vi "Discover ALL VIs in Memory.vi"(5 "Show Progress (T)":bool=TRUE, 6 "Filtered Paths":path[](array[path]), 7 "Search Clones Up To":i32=100, 8 "error in":errorcluster, 9 "Globals?":bool=TRUE, 10 "File Extension Filters":string[](array[string]), 11 "Application in":refnum<vi>) -> (0 "error out":errorcluster, 1 "VIs (including clones)":string[](array[string]), 3 "Application out":refnum<vi>)   [LabVIEW 2013, in "LVTM.lvlib"]
uses:
  LVTM.lvlib
  Clone VIs FG Enum.ctl
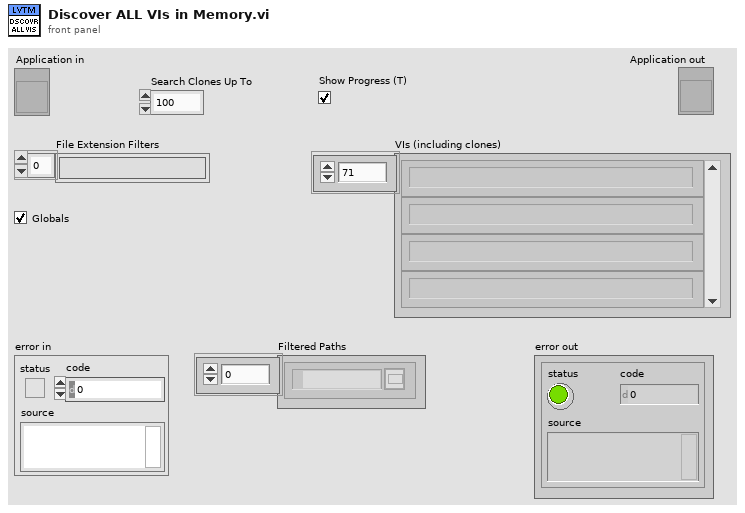
[diagram p1: front panel]
types:
  T1 = typedef "LVTM.lvlib/Clone VIs FG Enum.ctl" = enum16{"Get", "Get Active VIs", "Add VI"}
  T2 = enum32{"invalid VI type", "Standard VI", "Control VI", "Global VI", "Polymorphic VI", "Configuration VI", "SubSystem", "Facade VI", "Method VI", "Statechart Diagram VI"}
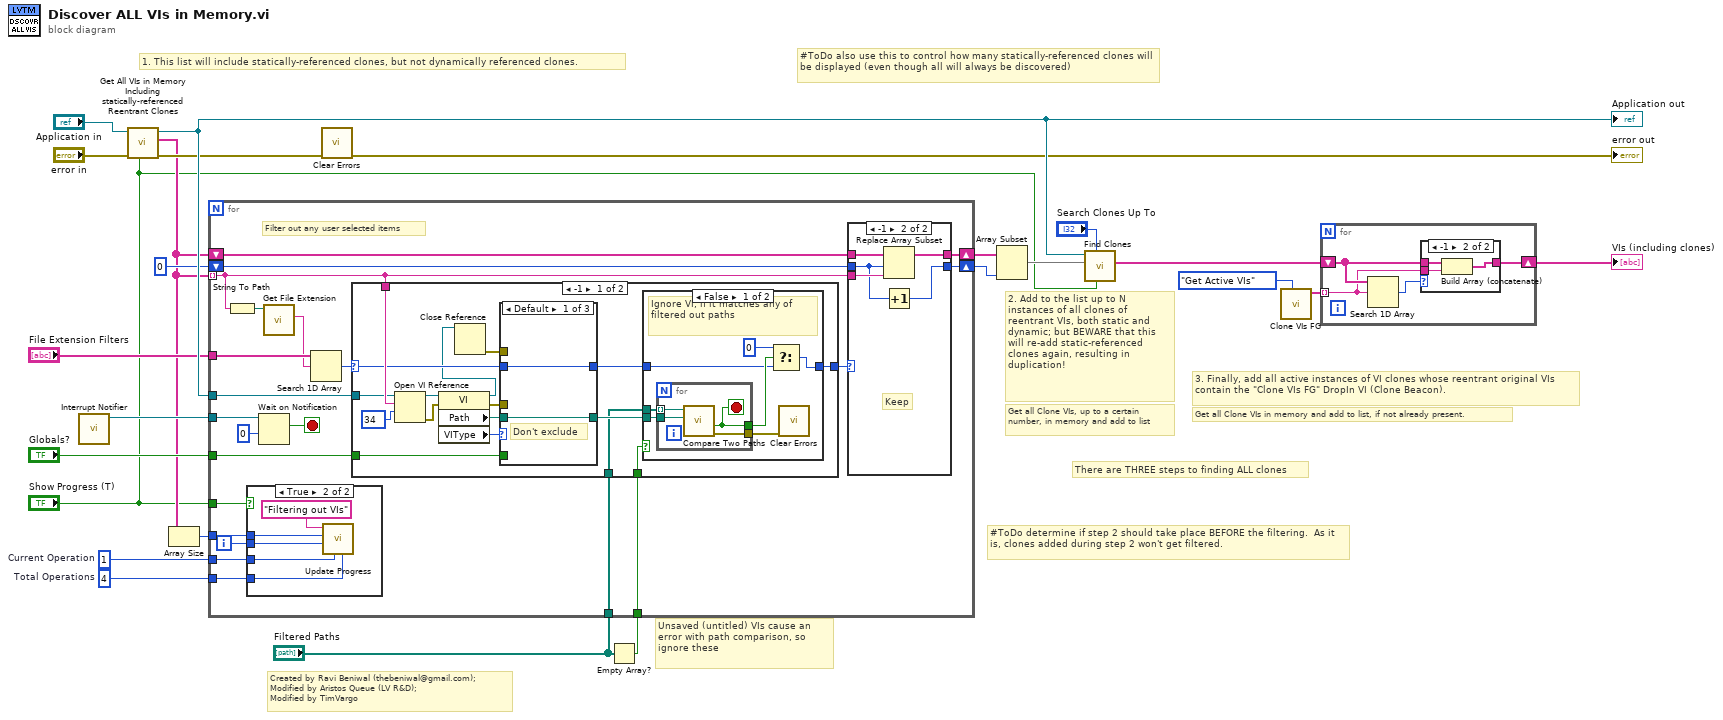
[diagram p0: block diagram]
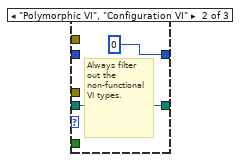
[diagram p5: hidden frame]
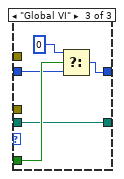
[diagram p6: hidden frame]
diagram:
  w2 = 4  # Total Operations
  w3 = 1  # Current Operation
  # "Unsaved (untitled) VIs cause an error with path comparison, so ignore these"
  # "#ToDo also use this to control how many statically-referenced clones will be displayed (even though all will always be discovered)"
  # "#ToDo determine if step 2 should take place BEFORE the filtering.  As it is, clones added during step 2 won't get filtered."
  # "2. Add to the list up to N instances of all clones of reentrant VIs, both static and dynamic; but BEWARE that this will re-add static-referenced clones again, resulting in duplication!"
  # "Get all Clone VIs, up to a certain \nnumber, in memory and add to list"
  # "1. This list will include statically-referenced clones, but not dynamically referenced clones."
  # "There are THREE steps to finding ALL clones"
  # "3. Finally, add all active instances of VI clones whose reentrant original VIs contain the \"Clone VIs FG\" DropIn VI (Clone Beacon)."
  # "Get all Clone VIs in memory and add to list, if not already present."
  # "Created by Ravi Beniwal (thebeniwal@gmail.com);\nModified by Aristos Queue (LV R&D);\nModified by TimVargo"
  n1 = call "Interrupt Notifier.vi"() -> ("Notifier out"=w6:refnum<notifier>)  [unwired: 10 in, 1 out]
  n2 = call "Get All VIs in Memory Including statically-referenced Reentrant Clones.vi"("Show Progress (T)"="Show Progress (T)", "error in (no error)"="error in", "App Refnum"="Application in") -> ("error out"=w16:errorcluster, "All VIs in Memory Including Reentrant Clones"=w5:string[], "App Refnum Out"=w24:refnum<vi>)  [unwired: 4 in, 2 out]
  "Application out" <- w24
  n3 = Array Size(array=w5) -> (size(s)=w4:i32)
  n4 = call <vilib>:"Clear Errors.vi"("error in (no error)"=w16) -> ("error out"=→"error out":errorcluster)  [unwired: 5 in, 1 out]
  n5 = Empty Array?(array="Filtered Paths") -> (empty?=w8:bool)
  n6 = for {
    tunnel: w5 -> [w37] mode=indexing
    tunnel: "File Extension Filters" -> [w45]
    shift-right: [w42] -> w11
    shift-left: w5 -> [w43]
    shift-right: [w40] -> w12
    shift-left: 0 -> [w41]
    tunnel: "Globals?" -> [w36]
    tunnel: w24 -> [w35]
    tunnel: w8 -> [w34]
    tunnel: "Filtered Paths" -> [w33]
    tunnel: w6 -> [w30]
    tunnel: w4 -> [w28]
    tunnel: w3 -> [w27]
    tunnel: w2 -> [w26]
    tunnel: "Show Progress (T)" -> [w25]
    i -> [w29]
    stop <- w31 stop-if-true
    # "Filter out any user selected items"
    n7 = String To Path(string=w37) -> (path=w46:path)
    n8 = case shown="True" w25 {
      tunnel: w29 -> [_ w51]
      tunnel: w28 -> [_ w50]
      tunnel: w27 -> [_ w48]
      tunnel: w26 -> [_ w47]
      frame False {
      }
      frame True {
        n9 = call "Update Progress.vi"("Total Operations (1)"=w47, "Current Operation (0)"=w48, "Current Iteration"=w51, "Total Interations"=w50, "Operation"="Filtering out VIs" ("Status")) -> ()  [unwired: 6 in, 1 out]
      }
    }
    n10 = Wait on Notification(notifier=w30, timeout in ms (-1)=0) -> (notification=w31:bool)  [unwired: 2 in, 3 out]
    n11 = call <vilib>:"Get File Extension.vi"("file"=w46) -> ("lowercase file extension"=w44:string)  [unwired: 6 in, 4 out]
    n12 = Search 1D Array(1D array=w45, element=w44) -> (index of element=w39:i32)  [unwired: 1 in]
    n13 = case shown="-1" w39 {
      selector: w39 -> [w65 w90]
      tunnel: [w60 w90] -> w38
      tunnel: w37 -> [w68 _]
      tunnel: w36 -> [w63 _]
      tunnel: w35 -> [w55 _]
      tunnel: w34 -> [w53 _]
      tunnel: w33 -> [w52 _]
      frame -1 {
        n14 = Open VI Reference(application reference (local)=w55, vi path=w68, options=34) -> (vi reference=w67:refnum<vi>, error out=w58:errorcluster)  [unwired: 3 in]
        n15 = property class="VI"(reference=w67, error in=w58) -> (reference out=w59:refnum<vi>, error out=w57:errorcluster, "Path"=w64:path, "VIType"=w66:T2)
        n16 = Close Reference(reference=w59) -> (error out=w56:errorcluster)  [unwired: 1 in]
        n17 = case shown="Default" w66 {
          tunnel: w65 -> [w82 _ w88]
          tunnel: [w82 0 ("index of element") w87] -> w61
          tunnel: w64 -> [w81 w83 w85]
          tunnel: w63 -> [_ _ w89]
          tunnel: [w81 w83 w85] -> w62
          tunnel: w57 -> [_ _ _]
          tunnel: w56 -> [_ _ _]
          frame Default {
            # "Don't exclude"
          }
          frame "Polymorphic VI", "Configuration VI" {
            # "Always filter out the non-functional VI types."
          }
          frame "Global VI" {
            n18 = Select(t=0, s=w89, f=w88) -> (s? t:f=w87:i32)
          }
        }
        n19 = case shown="False" w53 {
          tunnel: w62 -> [w75 _]
          tunnel: w61 -> [w73 w80]
          tunnel: [w71 w80] -> w60
          tunnel: w52 -> [w69 _]
          frame False {
            # "Ignore VI, if it matches any of filtered out paths"
            n20 = for {
              tunnel: w75 -> [w79]
              tunnel: [w76] -> w74
              tunnel: [w78] -> w70
              tunnel: w69 -> [w77] mode=indexing
              stop <- w76 stop-if-true
              n21 = call <vilib>:"Compare Two Paths.vi"("Path 2"=w79, "Path 1"=w77) -> ("error out"=w78:errorcluster, "Path 2 Relative to Path 1?"=w76:bool)  [unwired: 6 in, 2 out]
            }
            n22 = Select(t=0, s=w74, f=w73) -> (s? t:f=w71:i32)
            n23 = call <vilib>:"Clear Errors.vi"("error in (no error)"=w70) -> ()  [unwired: 5 in, 2 out]
          }
          frame True {
            # "Don't exclude items in vi.lib"
          }
        }
      }
      frame Default {
      }
    }
    n24 = case shown="-1" w38 {
      tunnel: w43 -> [w92 w97]
      tunnel: [w92 w96] -> w42
      tunnel: w37 -> [_ w95]
      tunnel: w41 -> [w91 w94]
      tunnel: [w91 w93] -> w40
      frame 0, Default {
        # "Discard"
      }
      frame -1 {
        # "Keep"
        n25 = Replace Array Subset(array=w97, new element=w95, index=w94) -> (w96:string[])
        n26 = Increment(x=w94) -> (x+1=w93:i32)
      }
    }
  }
  n27 = Array Subset(array=w11, length=w12) -> (w14:string[])  [unwired: 1 in]
  n28 = call "Find Clones.vi"("Show Progress (T)"="Show Progress (T)", "Search Clones Up To"="Search Clones Up To", "VIs in"=w14, "Application in"=w24) -> ("VIs (including clones) out"=w20:string[])  [unwired: 7 in]
  n29 = call "Clone VIs FG.vi"("Action (Add VI)"=Clone_VIs_FG_Enum."Get Active VIs" ("Action")) -> ("VIs"=w19:string[])  [unwired: 9 in, 1 out]
  n30 = for {
    shift-right: [w100] -> w21
    shift-left: w20 -> [w101]
    tunnel: w19 -> [w99] mode=indexing
    n31 = Search 1D Array(1D array=w101, element=w99) -> (index of element=w98:i32)  [unwired: 1 in]
    n32 = case shown="-1" w98 {
      tunnel: w101 -> [w102 w105]
      tunnel: [w102 w104] -> w100
      tunnel: w99 -> [_ w103]
      frame 0, Default {
      }
      frame -1 {
        n33 = Build Array (concatenate)(w105, w103) -> (w104:string[])
      }
    }
  }
  "VIs (including clones)" <- w21
